vi "读取字符串.vi"(8 "error in (no error)":errorcluster caption="错误输入（无错误）", 11 "串口 输入":refnum<class "串口.lvclass"> caption="DNL_LabVIEW Object in") -> (0 "error out":errorcluster caption="错误输出", 2 "字符串":string, 3 "串口 输出":refnum<class "串口.lvclass"> caption="DNL_LabVIEW Object out")   [LabVIEW 2012, in "串口.lvclass"]
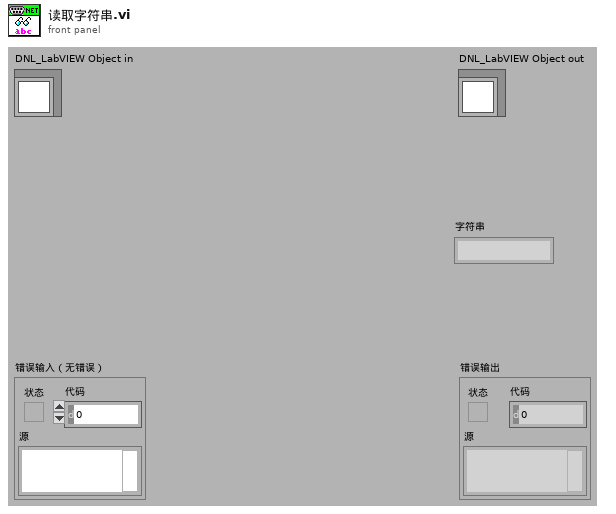
[diagram p1: front panel]
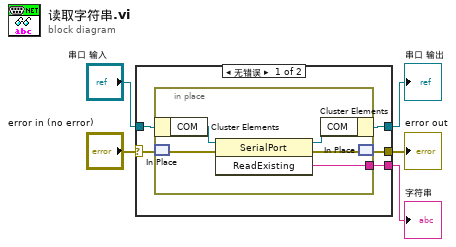
[diagram p0: block diagram]
diagram:
  n1 = case shown="无错误" "error in (no error)" {
    selector: "error in (no error)" -> [w10 w17]
    tunnel: [w6 w17] -> w4
    tunnel: [w7 w16] -> w2
    tunnel: "串口 输入" -> [w9 w16]
    tunnel: [w8 _] -> w1
    frame No Error {
      n2 = in-place {
        in-place-border: [w12] -> w8
        n3 = in-place-cluster #1(w9) -> ("COM"=w15:refnum<k24>)
        n4 = in-place-match #2(w10) -> (w14:errorcluster)
        n5 = invoke class="SerialPort" method="ReadExisting"(reference=w15, error in=w14) -> (reference out=w13:refnum<k24>, error out=w11:errorcluster, "ReadExisting"=w12:string)  [unwired: 1 in]
        n6 = in-place-cluster #1("COM"=w13) -> (w7:refnum<class "串口.lvclass">)
        n7 = in-place-match #2(w11) -> (w6:errorcluster)
      }
    }
    frame Error {
    }
  }
  "error out" <- w4
  "串口 输出" <- w2
  "字符串" <- w1
